vi "Set Value of LabVIEW Cluster.vi"(8 "error in (no error)":errorcluster, 10 "LabVIEW Cluster":refnum<vi>, 11 "JSON Tree Object":variant) -> (0 "error out":errorcluster)   [LabVIEW 2014, in "i3-json.lvlib"]
doc: "This VI takes a JSON Node (all types besides JSON Object) and assigns the value to the LabVIEW Base Type of compatible reference.\n\nIf the LabVIEW base type is an array of boolean, numeric, or string this function will attempt to check if a JSON Array type will map"
uses:
  i3-json.lvlib
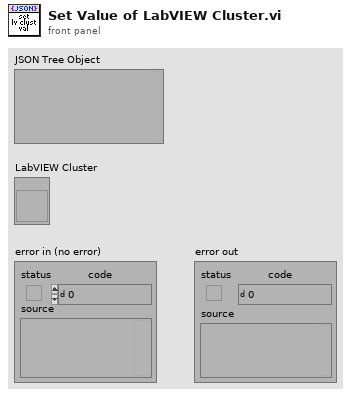
[diagram p1: front panel]
types:
  T1 = enum8{"Invalid Type", "Void", "I8", "I16", "I32", "I64", "U8", "U16", "U32", "U64", "Single Float", "Double Float", "Extended Float", "Single Complex", "Double Complex", "Extended Complex", "Enum U8", "Enum U16", "Enum U32", "Enum U64", "Single Float With Unit", "Double Float With Unit", "Extended Float With Unit", "Single Complex with Unit", "Double Complex with Unit", "Extended Complex with Unit", "Boolean", "String", "Path", "Picture", "Tag", "Array", "Cluster", "Variant", "LV Variant", "Waveform", "Timestamp", "Digital Waveform", "Digital Data", "ExpressData", "Refnum", "External Data", "VI", "Poly VI", "LabVIEW Class Instance", "Fixed Point"}
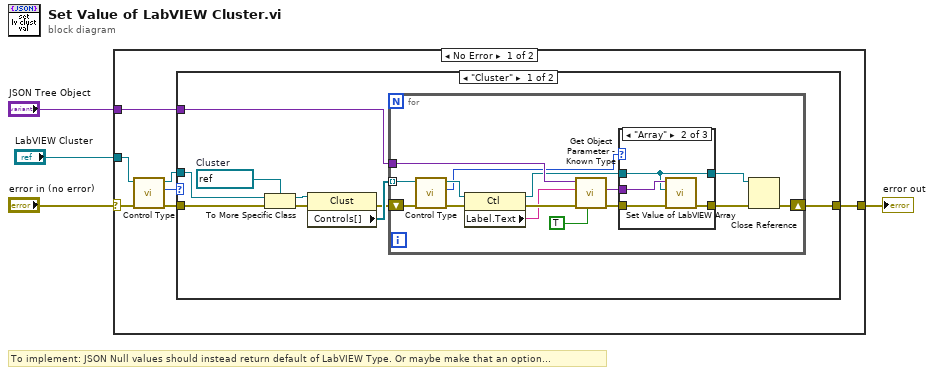
[diagram p0: block diagram]
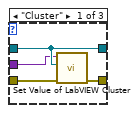
[diagram p2: hidden frame]
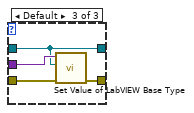
[diagram p3: hidden frame]
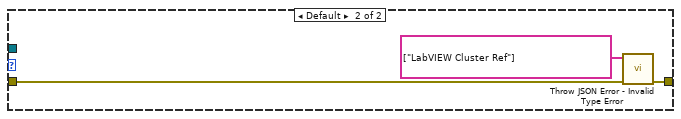
[diagram p4: hidden frame]
diagram:
  # "To implement: JSON Null values should instead return default of LabVIEW Type. Or maybe make that an option..."
  n1 = case shown="No Error" "error in (no error)" {
    selector: "error in (no error)" -> [w11 w51]
    tunnel: "LabVIEW Cluster" -> [w10 _]
    tunnel: "JSON Tree Object" -> [w7 _]
    tunnel: [w5 w51] -> w1
    frame No Error {
      n2 = call "Control Type.vi"("error in (no error)"=w11, "Control in"=w10) -> ("error out"=w6:errorcluster, "Type"=w9:T1, "Control out"=w8:refnum<vi>)  [unwired: 7 in]
      n3 = case shown="\"Cluster\"" w9 {
        tunnel: w8 -> [w19 _]
        tunnel: w7 -> [w13 _]
        tunnel: w6 -> [w20 w49]
        tunnel: [w12 w48] -> w5
        frame "Cluster" {
          w17 = refnum<vi> refnum  # Cluster
          n4 = To More Specific Class(target class=w17, reference=w19, error in=w20) -> (specific class reference=w16:refnum<vi>, error out=w18:errorcluster)
          n5 = property class="Clust"(reference=w16, error in=w18) -> (error out=w14:errorcluster, "Controls[]"=w15:refnum<vi>[])  [unwired: 1 out]
          n6 = for {
            tunnel: w15 -> [w34] mode=indexing
            tunnel: w13 -> [w31]
            shift-right: [w23] -> w12
            shift-left: w14 -> [w35]
            n7 = call "Control Type.vi"("error in (no error)"=w35, "Control in"=w34) -> ("error out"=w32:errorcluster, "Type"=w25:T1, "Control out"=w33:refnum<vi>)  [unwired: 7 in]
            n8 = property class="Ctl"(reference=w33, error in=w32) -> (reference out=w26:refnum<vi>, error out=w30:errorcluster, "Label.Text"=w29:string)
            n9 = call "Get Object Parameter - Known Type.vi"("Get Value as JSON Tree? (F)"=TRUE, "error in (no error)"=w30, "Parameter Name"=w29, "JSON Tree In (JSON Object)"=w31) -> ("error out"=w28:errorcluster, "Value"=w27:variant)  [unwired: 2 in, 4 out]
            n10 = case shown="\"Array\"" w25 {
              tunnel: [w39 w42 w45] -> w24
              tunnel: w28 -> [w38 w43 w47]
              tunnel: w27 -> [w36 w41 w46]
              tunnel: w26 -> [w37 w40 w44]
              tunnel: [w37 w40 w44] -> w22
              frame "Cluster" {
                n11 = call "Set Value of LabVIEW Cluster.vi"("error in (no error)"=w38, "LabVIEW Cluster"=w37, "JSON Tree Object"=w36) -> ("error out"=w39:errorcluster)  [unwired: 8 in]
              }
              frame "Array" {
                n12 = call "Set Value of LabVIEW Array.vi"("error in (no error)"=w43, "LabVIEW Array"=w40, "JSON Tree Array"=w41) -> ("error out"=w42:errorcluster)  [unwired: 8 in]
              }
              frame Default {
                n13 = call "Set Value of LabVIEW Base Type.vi"("error in (no error)"=w47, "LabVIEW Base Type"=w44, "JSON Tree Node"=w46) -> ("error out"=w45:errorcluster)  [unwired: 8 in]
              }
            }
            n14 = Close Reference(reference=w22, error in (no error)=w24) -> (error out=w23:errorcluster)
          }
        }
        frame Default {
          n15 = call "Throw JSON Error - Invalid Type Error.vi"("error in (no error)"=w49, "Valid Types"=string[] ["LabVIEW Cluster Ref"]) -> ("error out"=w48:errorcluster)  [unwired: 9 in]
        }
      }
    }
    frame Error {
    }
  }
  "error out" <- w1
